vi "AngleModulus_Example.vi"() -> ()   [LabVIEW 2019]
uses:
  <vilib>/Rock Robotics/WPI/ThirdParty/JAS_Junk/TrajLib/MathUtil_InputModulus.vi
  <vilib>/Rock Robotics/WPI/ThirdParty/JAS_Junk/TrajLib/Trajectory_Library.lvlib
panel:
  out "Angle Moduls\nRadians":dbl format="%15.3f"
  in  "Input":dbl(slide)=-0.015748031496062964 scale=-30.0..30.0
  out "Angle Modulus Trend":cluster{"Input":dbl, "Result":dbl}(graph)
  out "Raw Angle\nRadians":dbl=10.0 format="%15.3f"
  # "Analog  - Angle Modulus - Example"
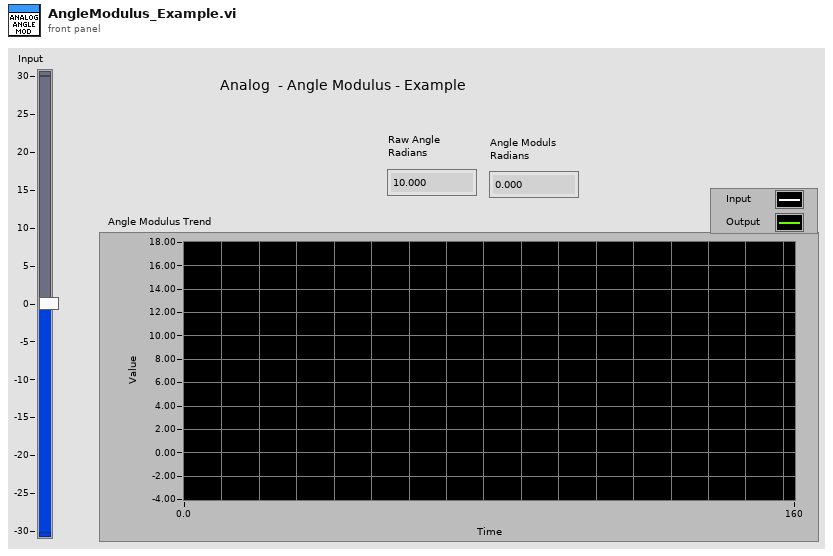
[diagram p1: front panel]
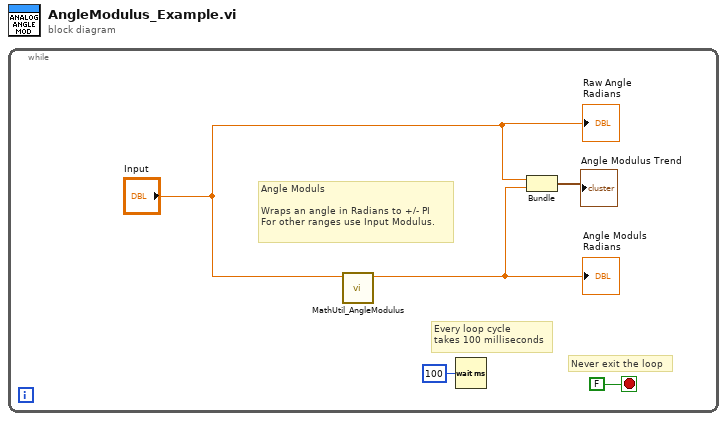
[diagram p0: block diagram]
diagram:
  n1 = while {
    stop <- FALSE stop-if-true
    # "Angle Moduls\n\nWraps an angle in Radians to +/- PI\nFor other ranges use Input Modulus."
    # "Every loop cycle\ntakes 100 milliseconds"
    # "Never exit the loop"
    n2 = call <vilib>:"MathUtil_AngleModulus.vi"("InputAngle"="Input") -> ("ModulsAngle"=w1:dbl)  [unwired: 10 in]
    "Angle Moduls\nRadians" <- w1
    n3 = Wait (ms)(milliseconds to wait=u32 100) -> ()  [unwired: 1 out]
    n4 = Bundle("Input"="Input", "ModulsAngle"=w1) -> (→"Angle Modulus Trend":cluster{"Input":dbl, "ModulsAngle":dbl})  [unwired: 1 in]
    "Raw Angle\nRadians" <- "Input"
  }
